vi "ep_Check RVC Settings.vi"(8 "error in (no error)":errorcluster, 11 "RVC settings":T1={"min rate of change [%/s]"=0.5, "steadiness of steady state [%]"=0.2, "min steady state duration [s]"=1.0, "min steady state difference [%]"=0.0, "max voltage change [%]"=3.3}) -> (0 "error out":errorcluster)   [LabVIEW 2014, in "NI_EP_Power Quality.lvlib"]
uses:
  <vilib>/addons/Electrical Power/PQ/NI_EP_Power Quality.lvlib
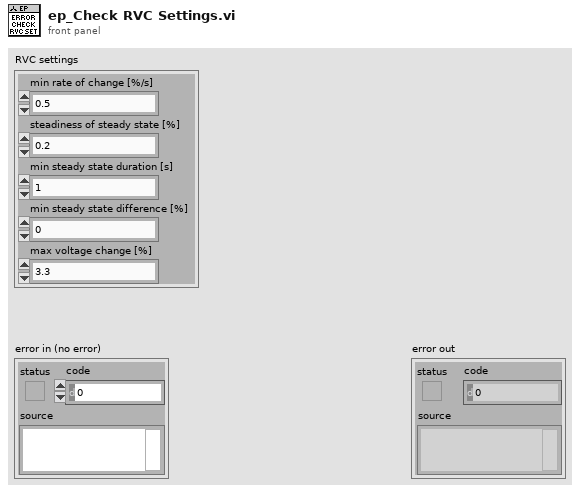
[diagram p1: front panel]
types:
  T1 = cluster{"min rate of change [%/s]":dbl, "steadiness of steady state [%]":dbl, "min steady state duration [s]":dbl, "min steady state difference [%]":dbl, "max voltage change [%]":dbl}
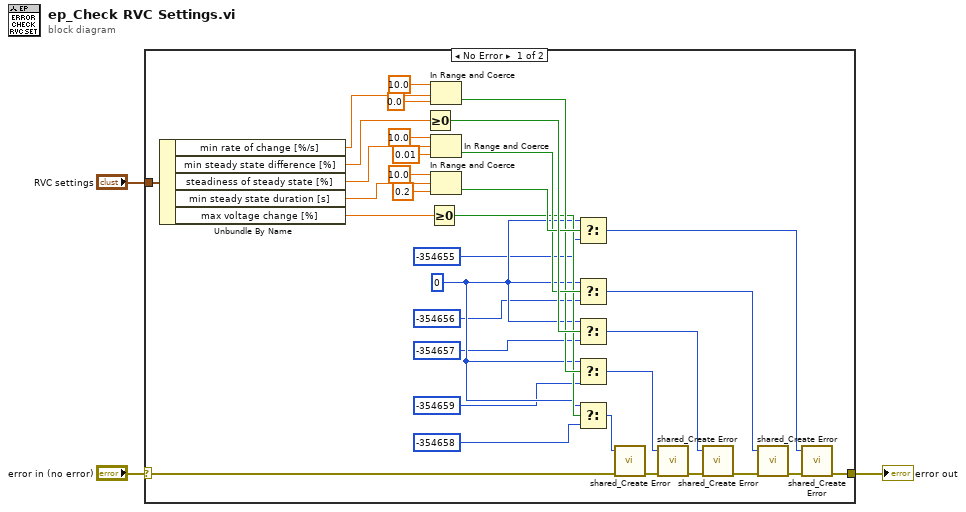
[diagram p0: block diagram]
diagram:
  n1 = case shown="No Error" "error in (no error)" {
    selector: "error in (no error)" -> [w5 w38]
    tunnel: "RVC settings" -> [w24 _]
    tunnel: [w4 w38] -> w1
    frame No Error {
      w20 = 0 ("error code (0)")
      n2 = Unbundle By Name(w24) -> ("min rate of change [%/s]"=w27:dbl, "min steady state difference [%]"=w36:dbl, "steadiness of steady state [%]"=w28:dbl, "min steady state duration [s]"=w33:dbl, "max voltage change [%]"=w22:dbl)
      n3 = Greater Or Equal To 0?(x=w36) -> (x >= 0?=w37:bool)
      n4 = Greater Or Equal To 0?(x=w22) -> (x >= 0?=w21:bool)
      n5 = In Range and Coerce(upper limit=10.0, x=w27, lower limit=0.0) -> (In Range?=w25:bool)  [unwired: 1 out]
      n6 = In Range and Coerce(upper limit=10.0, x=w28, lower limit=0.01) -> (In Range?=w31:bool)  [unwired: 1 out]
      n7 = In Range and Coerce(upper limit=10.0, x=w33, lower limit=0.2) -> (In Range?=w34:bool)  [unwired: 1 out]
      n8 = Select(t=w20, s=w34, f=-354655 ("error code (0)")) -> (s? t:f=w7:i32)
      n9 = Select(t=w20, s=w31, f=-354656 ("error code (0)")) -> (s? t:f=w10:i32)
      n10 = Select(t=w20, s=w37, f=-354657 ("error code (0)")) -> (s? t:f=w13:i32)
      n11 = Select(t=w20, s=w25, f=-354659 ("error code (0)")) -> (s? t:f=w15:i32)
      n12 = Select(t=w20, s=w21, f=-354658 ("error code (0)")) -> (s? t:f=w18:i32)
      n13 = call <vilib>:"shared_Create Error.vi"("error in (no error)"=w5, "error code (0)"=w18) -> ("error out"=w16:errorcluster)  [unwired: 9 in]
      n14 = call <vilib>:"shared_Create Error.vi"("error in (no error)"=w16, "error code (0)"=w15) -> ("error out"=w12:errorcluster)  [unwired: 9 in]
      n15 = call <vilib>:"shared_Create Error.vi"("error in (no error)"=w12, "error code (0)"=w13) -> ("error out"=w9:errorcluster)  [unwired: 9 in]
      n16 = call <vilib>:"shared_Create Error.vi"("error in (no error)"=w9, "error code (0)"=w10) -> ("error out"=w6:errorcluster)  [unwired: 9 in]
      n17 = call <vilib>:"shared_Create Error.vi"("error in (no error)"=w6, "error code (0)"=w7) -> ("error out"=w4:errorcluster)  [unwired: 9 in]
    }
    frame Error {
    }
  }
  "error out" <- w1
